vi "release queue.vi"(8 "error in (no error)":errorcluster, 11 "Queue in":refnum<queue>) -> (0 "error out":errorcluster)   [LabVIEW 2024, in "ED Queued State Machine.lvlib"]
uses:
  ED Queued State Machine.lvlib
  state and data--cluster.ctl
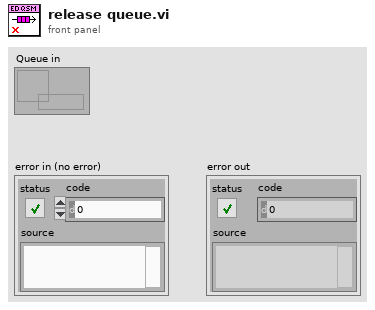
[diagram p1: front panel]
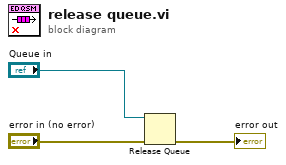
[diagram p0: block diagram]
diagram:
  n1 = Release Queue(queue="Queue in", error in (no error)="error in (no error)") -> (error out=→"error out":errorcluster)  [unwired: 1 in, 2 out]
